vi "Get Instr Identifier.vi"(8 "error in":errorcluster, 11 "Configuration Base in":refnum<class "CFG JSON.lvclass">) -> (0 "error out":errorcluster, 2 "Instr Ident":string, 3 "Configuration Base out":refnum<class "CFG JSON.lvclass">)   [LabVIEW 2023, in "HAL GOOP4.lvlib" / "CFG JSON.lvclass"]
uses:
  CFG JSON.lvclass
  CFG JSON.lvclass/CFG JSON.ctl
  5ee9908e-5bcb-4a27-ad9d-9e265a0da21d.vi
  5ee9908e-5bcb-4a27-ad9d-9e265a0da21d.vi/a4169a97-72fc-4003-a778-603cf20cafa0.vi
  <vilib>/JDP Science/JSONtext/Find Item.vi
  <vilib>/JDP Science/JSONtext/Next JSON Value.vi
  <vilib>/JDP Science/JSONtext/String Subset.vi
  <vilib>/JDP Science/JSONtext/Parsing/Advance past next JSON Value (inlined COPY).vi
  <vilib>/JDP Science/JSONtext/Parsing/Advance past whitespace.vi
  <vilib>/JDP Science/JSONtext/Parsing/Advance past String.vi
  <vilib>/JDP Science/JSONtext/Parsing/Advance past Number.vi
  <vilib>/JDP Science/JSONtext/Parsing/Advance past Line Ending.vi
  <vilib>/JDP Science/JSONtext/Parsing/Parse Full Path or Item Name.vi
  <vilib>/JDP Science/JSONtext/Parsing/Advance past Array.vi
  <vilib>/JDP Science/JSONtext/Parsing/Advance past Object.vi
  <vilib>/JDP Science/JSONtext/support/Error Cluster From Code.vi
  <vilib>/JDP Science/JSONtext/Offset/Find Item Locations by Path.vi
  <vilib>/JDP Science/JSONtext/JSON text to Variant.vi
  <vilib>/Utility/error.llb/Error Cluster From Error Code.vi
  <vilib>/JDP Science/JSONtext/LVClass Serializer/JSONtext LVClass Serializer.lvclass
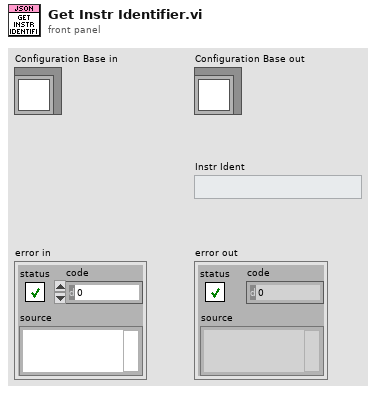
[diagram p1: front panel]
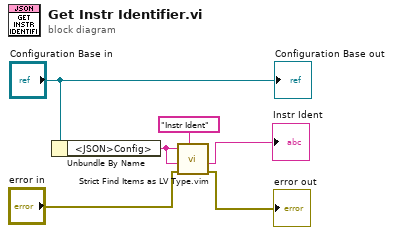
[diagram p0: block diagram]
diagram:
  n1 = Unbundle By Name("Configuration Base in") -> ("<JSON>Config>"=w3:string)
  n2 = call "Strict Find Items as LV Type.vim"("$Path or Item Name"="Instr Ident", "error in"="error in", "Data Type and Default Value"=w3, "JSON"=w3) -> ("error out"=→"error out":errorcluster, "Data out"=→"Instr Ident":string)  [unwired: 6 in]
  "Configuration Base out" <- "Configuration Base in"
